vi "[GV]_BRAKE.vi"() -> ()   [LabVIEW 2016]
panel:
  in  "BRAKE":u16
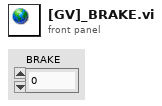
[diagram p1: front panel]
diagram:
